vi "GE 5565PIORC.PIO.Write (Bool).vi"(8 "error in (no error)":errorcluster, 9 "data":bool, 10 "offset":u32, 11 "GE 5565PIORC in":refnum<class "GE 5565PIORC.lvclass">) -> (0 "error out":errorcluster, 1 "data out":bool, 3 "GE 5565PIORC out":refnum<class "GE 5565PIORC.lvclass">)   [LabVIEW 2017, in "GE 5565PIORC.lvclass"]
doc: "Writes the contents of <B>data</B> to the specified <B>offset</B>."
uses:
  GE 5565PIORC.lvclass
  <vilib>/Instr/_visa.llb/VISA Register Access Address Space.ctl
  GE 5565PIORC.lvclass/GE 5565PIORC.ctl
  GE 5565PIORC.VISA.Move Out.String (U8).vi
  GE 5565PIORC.VISA.Return Handler.vi
  <vilib>/Utility/error.llb/Error Cluster From Error Code.vi
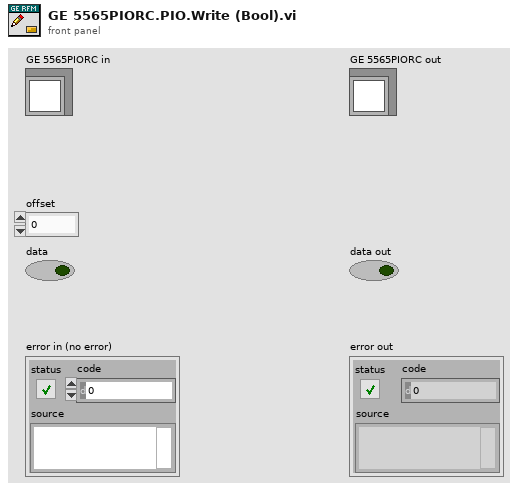
[diagram p1: front panel]
types:
  T1 = typedef "VISA Register Access Address Space.ctl" = u16
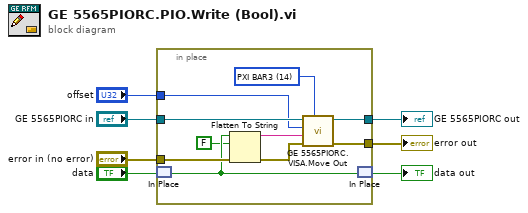
[diagram p0: block diagram]
diagram:
  n1 = in-place {
    in-place-border: "error in (no error)" -> [w15]
    in-place-border: [w13] -> w6
    in-place-border: "GE 5565PIORC in" -> [w16]
    in-place-border: "offset" -> [w11]
    in-place-border: [w10] -> w1
    w17 = T1 14 items=["VXI/VME A16"=1, "VXI/VME A24"=2, "VXI/VME A32"=3, "VXI/VME A64"=4, "PXI Memory Allocations"=9, "PXI Configuration"=10, "PXI BAR0"=11, "PXI BAR1"=12, "PXI BAR2"=13, "PXI BAR3"=14, "PXI BAR4"=15, "PXI BAR5"=16] ("address space")
    n2 = in-place-match #1("data") -> (w9:bool)
    n3 = Flatten To String(anything=w9, prepend array or string size? (T)=FALSE, error in (no error)=w15) -> (data string=w12:string, error out=w14:errorcluster)  [unwired: 1 in, 1 out]
    n4 = call-poly "GE 5565PIORC.VISA.Move Out.vi"("address space"=w17, "error in (no error)"=w14, "data in"=w12, "offset"=w11, "GE 5565PIORC in"=w16) -> ("error out"=w13:errorcluster, "GE 5565PIORC out"=w10:refnum<class "GE 5565PIORC.lvclass">)  [unwired: 4 in, 1 out]
    n5 = in-place-match #1(w9) -> (→"data out":bool)
  }
  "GE 5565PIORC out" <- w1
  "error out" <- w6
